vi "Control Alogrithm.vi"(10 "output cluster":cluster{"upper limit":dbl, "lower limit":dbl}, 11 "Voltage Feedback":dbl) -> (0 "In Range?":bool, 1 "voltage lower":bool, 2 "voltage higher":bool, 3 "Case":u32, 5 "output cluster 2":cluster{"upper limit":dbl, "lower limit":dbl})   [LabVIEW 2019]
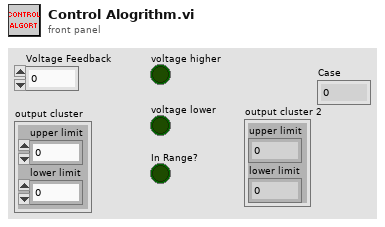
[diagram p1: front panel]
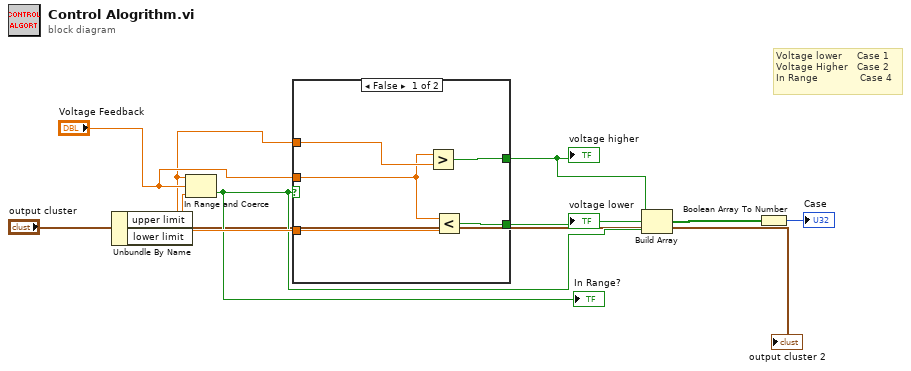
[diagram p0: block diagram]
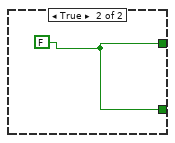
[diagram p2: hidden frame]
diagram:
  # "Voltage lower     Case 1\nVoltage Higher   Case 2 \nIn Range              Case 4"
  n1 = Unbundle By Name("output cluster") -> ("upper limit"=w7:dbl, "lower limit"=w8:dbl)
  n2 = In Range and Coerce(upper limit=w7, x="Voltage Feedback", lower limit=w8) -> (In Range?=w4:bool)  [unwired: 1 out]
  "In Range?" <- w4
  n3 = case shown="False" w4 {
    tunnel: w7 -> [w14 _]
    tunnel: w8 -> [w13 _]
    tunnel: "Voltage Feedback" -> [w12 _]
    tunnel: [w11 w15] -> w5
    tunnel: [w10 w15] -> w6
    frame False {
      n4 = Greater?(x=w12, y=w14) -> (0:w10:bool)
      n5 = Less?(x=w12, y=w13) -> (x < y?=w11:bool)
    }
    frame True {
      w15 = FALSE
    }
  }
  "voltage higher" <- w6
  "voltage lower" <- w5
  n6 = Build Array(w6, w5, w4) -> (w2:bool[])
  n7 = Boolean Array To Number(Boolean array=w2) -> (number=→"Case":u32)
  "output cluster 2" <- "output cluster"
